vi "Configure Session.vi"(8 "error in":errorcluster, 11 "Plugin in":refnum<class "Output Sequencer.lvclass">) -> (0 "error out":errorcluster, 3 "Plugin out":refnum<class "Output Sequencer.lvclass">)   [LabVIEW 2024, in "Output Sequencer.lvlib" / "Output Sequencer.lvclass"]
uses:
  Output Sequencer.lvclass
  C:/Program Files/National Instruments/LabVIEW 2024/vi.lib/FlexLogger/SDK/PluginSDK.lvlibp/PEFClasses/SDK/Plugin/Plugin.lvclass
  Types/Sequencer State.ctl
  Output Sequencer.lvclass/Output Sequencer.ctl
  <vilib>/FlexLogger/SDK/PluginSDK.lvlibp/PEFClasses/SDK/Producer Channel/Producer Channel.lvclass
  C:/Program Files/National Instruments/LabVIEW 2024/vi.lib/FlexLogger/SDK/PluginSDK.lvlibp/PEFClasses/SDK/Channel/Channel.lvclass
  Globals/Global Strings.vi
  <vilib>/FlexLogger/SDK/PluginSDK.lvlibp/PEFClasses/SDK/Plugin/ParameterAccess/Read String.vi
  <vilib>/FlexLogger/SDK/PluginSDK.lvlibp/PEFClasses/SDK/Plugin/Plugin.lvclass
  C:/Program Files/National Instruments/LabVIEW 2024/vi.lib/FlexLogger/SDK/PluginSDK.lvlibp/PEFClasses/SDK/Processing Element/Processing Element.lvclass
  C:/Dev/GitHub/ni/niflexlogger-plugins/PDK plugins/Output Sequencer/source/Output Sequencer/Output Sequencer.lvclass
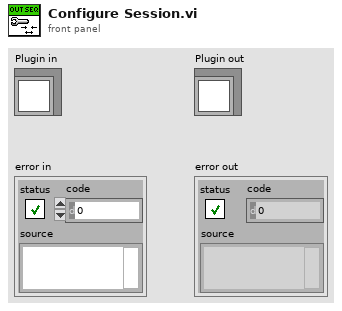
[diagram p1: front panel]
types:
  T1 = typedef "Output Sequencer.lvlib/Output Sequencer.lvclass/Sequencer State.ctl" = enum16{"Error", "Initialize", "Prepare channels", "Wait for test", "Wait for %.1f sec", "Wait for trigger", "Stop condition", "Wait for resume", "Running", "Paused", "No valid step", "Stopped"}
  T2 = typedef "Output Sequencer.lvlib/Settings UI.lvclass/Settings.ctl" = cluster{"Plug-in Version":string, "Step Values":T3[], "Only Execute When Test Running":bool, "Reset Sequence When Test Starts":bool, "Number of Sequence Steps":i32, "Num of Analog Channels":i32, "Num of Digital Channels":i32, "Delay Before Starting Sequence":dbl, "Default Analog Values":dbl[], "Default Digital Values":bool[], "Max Iterations":u32, "Use last value when stopped":bool, "Prioritize exact values":bool, "Enable advanced step timing":bool, "Enable step conditions":bool, "Show confirmation dialogs":bool, "Start condition":string, "Enable re-triggering":bool, "Stop condition":string}
  T3 = typedef "Output Sequencer.lvlib/Settings UI.lvclass/Step Settings.ctl" = cluster{"Description":string, "Precondition":string, "Duration":dbl, "Mode":string, "Delay Between Values":dbl, "Analog Values":string[], "Digital Values":string[], "Postcondition":string, "On True":string, "On False":string}
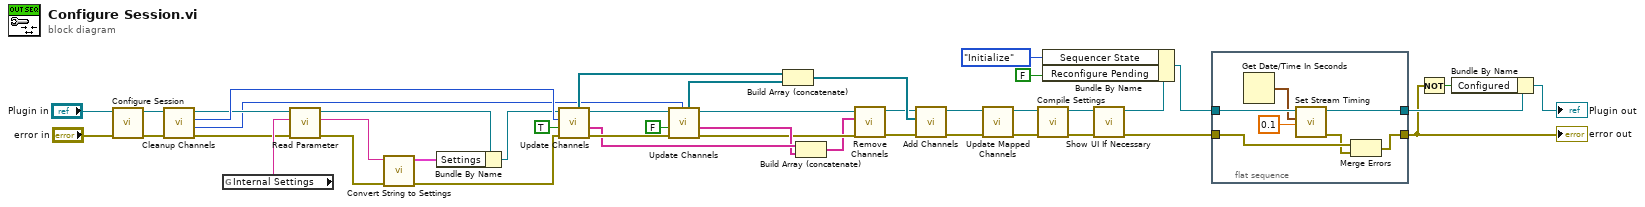
[diagram p0: block diagram]
diagram:
  n1 = call-parent "Configure Session.vi"("error in (no error)"="error in", "Processing Element in"="Plugin in") -> ("error out"=w31:errorcluster, "Processing Element out"=w27:refnum<class "Output Sequencer.lvclass">)  [unwired: 8 in]
  n2 = call "Cleanup Channels.vi"("error in (no error)"=w31, "Output Sequencer In"=w27) -> ("error out"=w28:errorcluster, "Num of Digital Channels"=w26:i32, "Num of Analog Channels"=w30:i32, "Output Sequencer out"=w29:refnum<class "Output Sequencer.lvclass">)  [unwired: 6 in]
  n3 = global read "Global Strings.vi" "Internal Settings"() -> (w39:string)
  n4 = call-poly <vilib>:"Read Parameter.vi"("error in (no error)"=w28, "Name"=w39, "Plugin in"=w29) -> ("error out"=w32:errorcluster, "Value"=w23:string, "Plugin out"=w22:refnum<class "Output Sequencer.lvclass">)  [unwired: 5 in, 1 out]
  n5 = call "Convert String to Settings.vi"("error in (no error)"=w32, "String In"=w23) -> ("error out"=w18:errorcluster, "Settings Out"=w20:T2)  [unwired: 8 in]
  n6 = Bundle By Name(cluster=w22, "Settings"=w20) -> (w19:refnum<class "Output Sequencer.lvclass">)
  n7 = call "Update Channels.vi"("error in (no error)"=w18, "Analog"=TRUE, "Previous Number of Channels"=w30, "Output Sequencer in"=w19) -> ("error out"=w41:errorcluster, "Channels to Remove"=w36:string[], "Output Sequencer out"=w17:refnum<class "Output Sequencer.lvclass">, "Channels to Add"=w38:refnum<class "Producer Channel.lvclass">[])  [unwired: 4 in]
  n8 = call "Update Channels.vi"("error in (no error)"=w41, "Analog"=FALSE, "Previous Number of Channels"=w26, "Output Sequencer in"=w17) -> ("error out"=w33:errorcluster, "Channels to Remove"=w35:string[], "Output Sequencer out"=w34:refnum<class "Output Sequencer.lvclass">, "Channels to Add"=w37:refnum<class "Producer Channel.lvclass">[])  [unwired: 4 in]
  n9 = Build Array (concatenate)(w38, w37) -> (w12:refnum<class "Producer Channel.lvclass">[])
  n10 = Build Array (concatenate)(w36, w35) -> (w11:string[])
  n11 = call-dynamic "Remove Channels.vi"("error in (no error)"=w33, "Unique Channel Identifiers to Delete"=w11, "Plugin in"=w34) -> ("error out"=w9:errorcluster, "Plugin out"=w10:refnum<class "Output Sequencer.lvclass">)  [unwired: 7 in]
  n12 = call <vilib>:"Add Channels.vi"("error in (no error)"=w9, "Channels"=w12, "Plugin in"=w10) -> ("error out"=w25:errorcluster, "Plugin out"=w24:refnum<class "Output Sequencer.lvclass">)  [unwired: 7 in]
  n13 = call "Update Mapped Channels.vi"("error in (no error)"=w25, "Output Sequencer in"=w24) -> ("error out"=w13:errorcluster, "Output Sequencer out"=w14:refnum<class "Output Sequencer.lvclass">)  [unwired: 8 in]
  n14 = call "Compile Settings.vi"("error in (no error)"=w13, "Plugin in"=w14) -> ("error out"=w5:errorcluster, "Plugin out"=w8:refnum<class "Output Sequencer.lvclass">)  [unwired: 8 in]
  n15 = call "Show UI If Necessary.vi"("error in (no error)"=w5, "Output Sequencer in"=w8) -> ("error out"=w6:errorcluster, "Output Sequencer out"=w7:refnum<class "Output Sequencer.lvclass">)  [unwired: 8 in]
  n16 = Bundle By Name(cluster=w7, "Sequencer State"=Sequencer_State."Initialize" ("State.Sequencer State"), "Reconfigure Pending"=FALSE) -> (w21:refnum<class "Output Sequencer.lvclass">)
  n17 = flat-sequence {
    tunnel: [w51] -> w4
    tunnel: [w47] -> w2
    tunnel: w21 -> [w50]
    tunnel: w6 -> [w46]
    frame #0 {
      n18 = Get Date/Time In Seconds ("t0")() -> (seconds since 1Jan1904=w49:timestamp)
      n19 = call-dynamic "Set Stream Timing.vi"("dt(sec)"=0.1 ("dt (sec)"), "Start Time"=w49, "Plugin in"=w50) -> ("error out"=w45:errorcluster, "Plugin out"=w51:refnum<class "Output Sequencer.lvclass">)  [unwired: 7 in]
      n20 = Merge Errors(w46, w45) -> (w47:errorcluster)
    }
  }
  n21 = Not(x=w2) -> (.not. x?=w1:bool)
  n22 = Bundle By Name(cluster=w4, "Configured"=w1) -> (→"Plugin out":refnum<class "Output Sequencer.lvclass">)
  "error out" <- w2
